vi "6704_set_static_voltages.vi"(6 "error in":errorcluster, 8 "6704 Static Voltage Settings":T1={"Device Name"="6704_Static", "Voltages"=[5.0, 0.0, 0.0, 0.0, 0.0, 0.0, 0.0, 0.0, 0.0, 0.0, 0.0, 0.0, 0.0, 0.0, 0.0, 0.0]}) -> (0 "error out":errorcluster, 2 "Voltages Out":dbl[](array[numeric]))   [LabVIEW 2013]
uses:
  6704_static_voltages_control.ctl
  6704_state_machine_enum.ctl
  <vilib>/DAQmx/write.llb/DAQmx Write (Analog 1D DBL NChan 1Samp).vi
  <vilib>/DAQmx/create/channels.llb/DAQmx Create Channel (AO-Voltage-Basic).vi
  <vilib>/DAQmx/miscellaneous.llb/DAQmx Fill In Error Info.vi
  <resource>/objmgr/daqmx.rc
panel:
  out "AO.Voltage.Rngs":dbl[](array[numeric])
  out "Active Device":tag
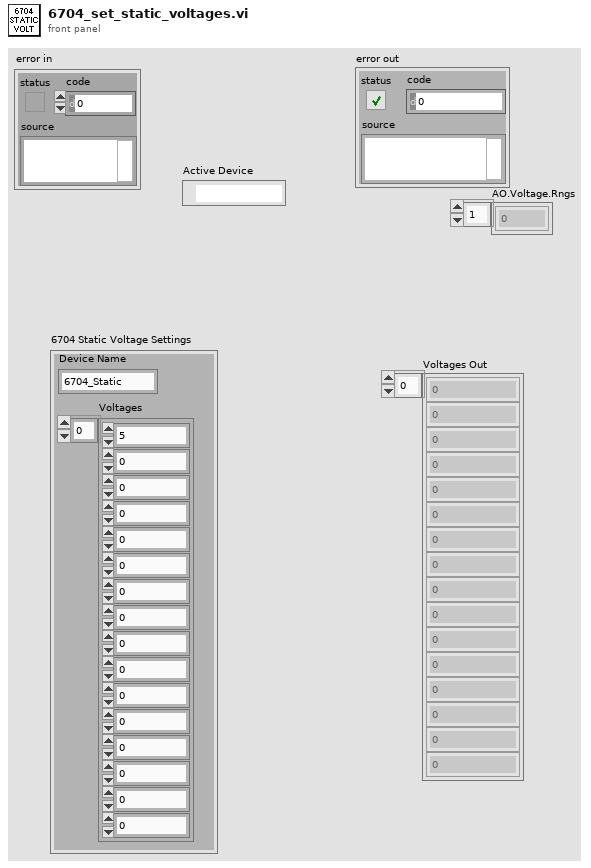
[diagram p1: front panel]
types:
  T1 = typedef "6704_static_voltages_control.ctl" = cluster{"Device Name":string, "Voltages":dbl[]}
  T2 = typedef "6704_state_machine_enum.ctl" = enum16{"Initialize", "Set Voltages", "Custom Voltages", "Debug"}
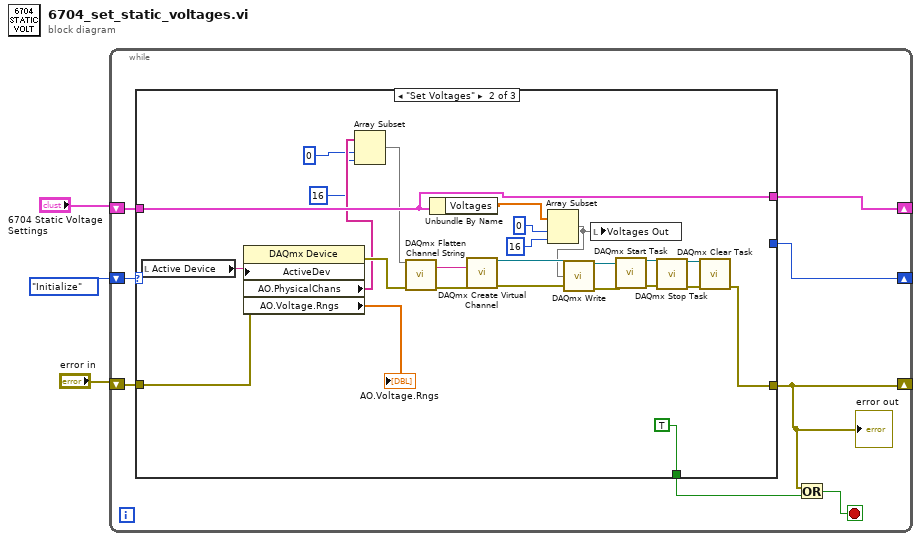
[diagram p0: block diagram]
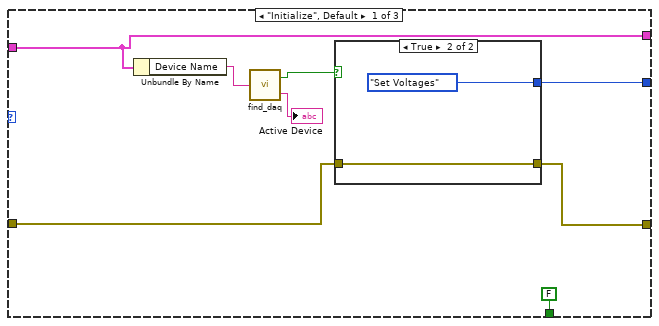
[diagram p2: hidden frame]
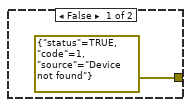
[diagram p3: hidden frame]
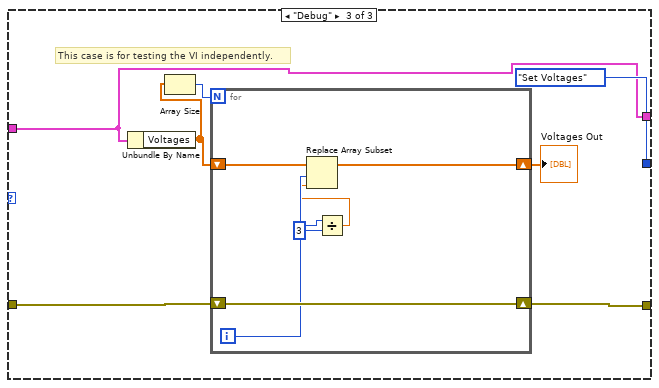
[diagram p4: hidden frame]
diagram:
  n1 = while {
    shift-right: [w4] -> _
    shift-left: "error in" -> [w9]
    shift-right: [w8] -> _
    shift-left: 6704_state_machine_enum."Initialize" -> [w11]
    shift-right: [w6] -> _
    shift-left: "6704 Static Voltage Settings" -> [w10]
    stop <- w7 stop-if-true
    n2 = case shown="\"Set Voltages\"" w11 {
      tunnel: w10 -> [w13 w38 w48]
      tunnel: w9 -> [w14 w47 w53]
      tunnel: [w16 _ 6704_state_machine_enum."Set Voltages"] -> w8
      tunnel: [w15 w41 w54] -> w4
      tunnel: [w13 w38 w48] -> w6
      tunnel: [FALSE ("y") TRUE ("y") _] -> w5
      frame "Initialize", Default {
        n3 = Unbundle By Name(w13) -> ("Device Name"=w19:string)
        n4 = call "find_daq.vi"("Device Name"=w19) -> ("Device Present"=w18:bool, "DAQmx Device Name"=→"Active Device":tag)
        n5 = case shown="True" w18 {
          tunnel: [_ 6704_state_machine_enum."Set Voltages"] -> w16
          tunnel: [errorcluster {"status"=TRUE, "code"=1, "source"="Device not found"} ("error in") w21] -> w15
          tunnel: w14 -> [_ w21]
          frame False {
          }
          frame True {
          }
        }
      }
      frame "Set Voltages" {
        n6 = local read "Active Device"() -> (w46:tag)
        n7 = property class="DAQmx Device"(error in=w47, "ActiveDev"=w46) -> (error out=w36:errorcluster, "AO.PhysicalChans"=w32:tag[], "AO.Voltage.Rngs"=→"AO.Voltage.Rngs":dbl[])  [unwired: 1 in, 1 out]
        n8 = Array Subset(array=w32, index=0, length=16) -> (w29:tag[])
        n9 = call <vilib>:"DAQmx Flatten Channel String.vi"("names in"=w29, "error in"=w36) -> ("names out"=w37:string, "error out"=w35:errorcluster)  [unwired: 12 in]
        n10 = Unbundle By Name(w38) -> ("Voltages"=w25:dbl[])
        n11 = call-poly <vilib>:"DAQmx Create Virtual Channel.vi"("physical channels"=w37, "error in"=w35) -> ("task out"=w28:refnum<k21>, "error out"=w45:errorcluster)  [unwired: 12 in]
        n12 = Array Subset(array=w25, index=0, length=16) -> (w24:dbl[])
        n13 = call-poly <vilib>:"DAQmx Write.vi"("task/channels in"=w28, "data"=w24, "error in"=w45) -> ("task out"=w44:refnum<k21>, "error out"=w43:errorcluster)  [unwired: 10 in, 1 out]
        n14 = local write "Voltages Out"(w24) -> ()
        n15 = call <vilib>:"DAQmx Start Task.vi"("task/channels in"=w44, "error in"=w43) -> ("task out"=w26:refnum<k21>, "error out"=w27:errorcluster)  [unwired: 12 in]
        n16 = call <vilib>:"DAQmx Stop Task.vi"("task/channels in"=w26, "error in"=w27) -> ("task out"=w40:refnum<k21>, "error out"=w42:errorcluster)  [unwired: 12 in]
        n17 = call <vilib>:"DAQmx Clear Task.vi"("task in"=w40, "error in"=w42) -> ("error out"=w41:errorcluster)  [unwired: 13 in]
      }
      frame "Debug" {
        # "This case is for testing the VI independently."
        n18 = Unbundle By Name(w48) -> ("Voltages"=w49:dbl[])
        n19 = Array Size(array=w49) -> (size(s)=w50:i32)
        n20 = for {
          N: w50 -> [_]
          shift-right: [w60] -> w54
          shift-left: w53 -> [w60]
          shift-right: [w58] -> w52
          shift-left: w49 -> [w59]
          i -> [w57]
          n21 = Divide(x=w57, y=3) -> (x/y=w55:dbl)
          n22 = Replace Array Subset(array=w59, new element=w55, index=w57) -> (w58:dbl[])
        }
        "Voltages Out" <- w52
      }
    }
    "error out" <- w4
    n23 = Or(x=w4, y=w5) -> (x .or. y?=w7:bool)
  }
